vi "set array to zero (dbl 1d).vi"(1 "array in":dbl[](array[numeric])) -> (0 "array out":dbl[](array[numeric]))   [LabVIEW 2012, in "common.lvlib"]
uses:
  common.lvlib
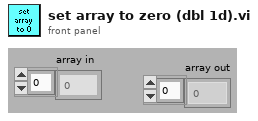
[diagram p1: front panel]
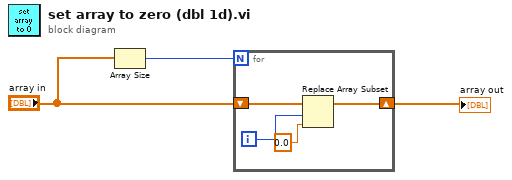
[diagram p0: block diagram]
diagram:
  n1 = Array Size(array="array in") -> (size(s)=w1:i32)
  n2 = for {
    N: w1 -> [_]
    shift-right: [w5] -> w2
    shift-left: "array in" -> [w7]
    i -> [w4]
    n3 = Replace Array Subset(array=w7, new element=0.0 ("new element/subarray"), index=w4) -> (w5:dbl[])
  }
  "array out" <- w2
